vi "Simple Delay Line.vi"() -> ()   [LabVIEW 2015]
uses:
  <vilib>/DAQmx/read.llb/DAQmx Read (Analog Wfm 1Chan NSamp).vi
  <vilib>/DAQmx/write.llb/DAQmx Write (Analog Wfm 1Chan NSamp).vi
  <vilib>/DAQmx/create/channels.llb/DAQmx Create Channel (AI-Voltage-Basic).vi
  <vilib>/DAQmx/create/channels.llb/DAQmx Create Channel (AO-Voltage-Basic).vi
  <vilib>/DAQmx/configure/timing.llb/DAQmx Timing (Sample Clock).vi
  <vilib>/DAQmx/configure/trigger.llb/DAQmx Reference Trigger (Analog Window).vi
  <vilib>/DAQmx/miscellaneous.llb/DAQmx Fill In Error Info.vi
  <resource>/objmgr/daqmx.rc
panel:
  in  "Speaker IR":path
  in  "Stimuli":dbl[](array[numeric])
  in  "Stimulus File":path=path "C:/Kate/matlabstim/IRs/testIR.mat"
  out "Now Playing":dbl=3.0
  out "data 2":waveform(dbl)(graph) caption="Stim"
  out "data":waveform(dbl)(graph)={"t0"=timestamp(3665351973.137573 s since 1904-01-01), "dt"=3.999999999999989e-06, "Y"=array[1250 elements], "attributes"=variant("NI_ChannelName"=variant(string "PXI1Slot2/ai1"), "NI_UnitDescription"=variant(string "Volts"))} caption="Call"
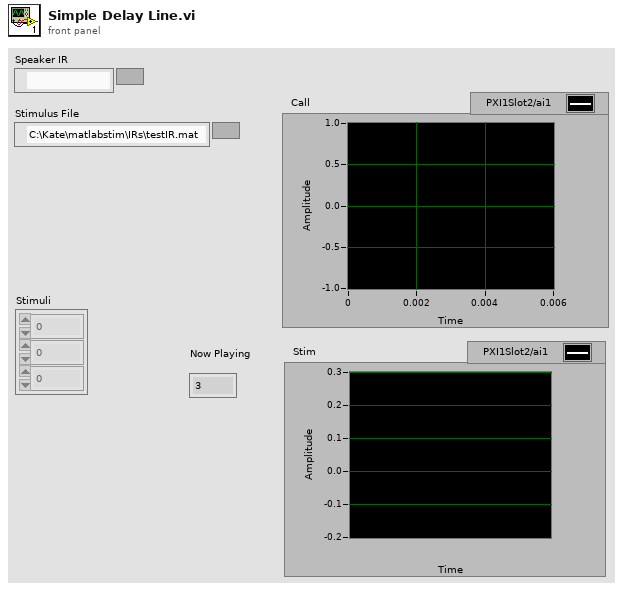
[diagram p1: front panel]
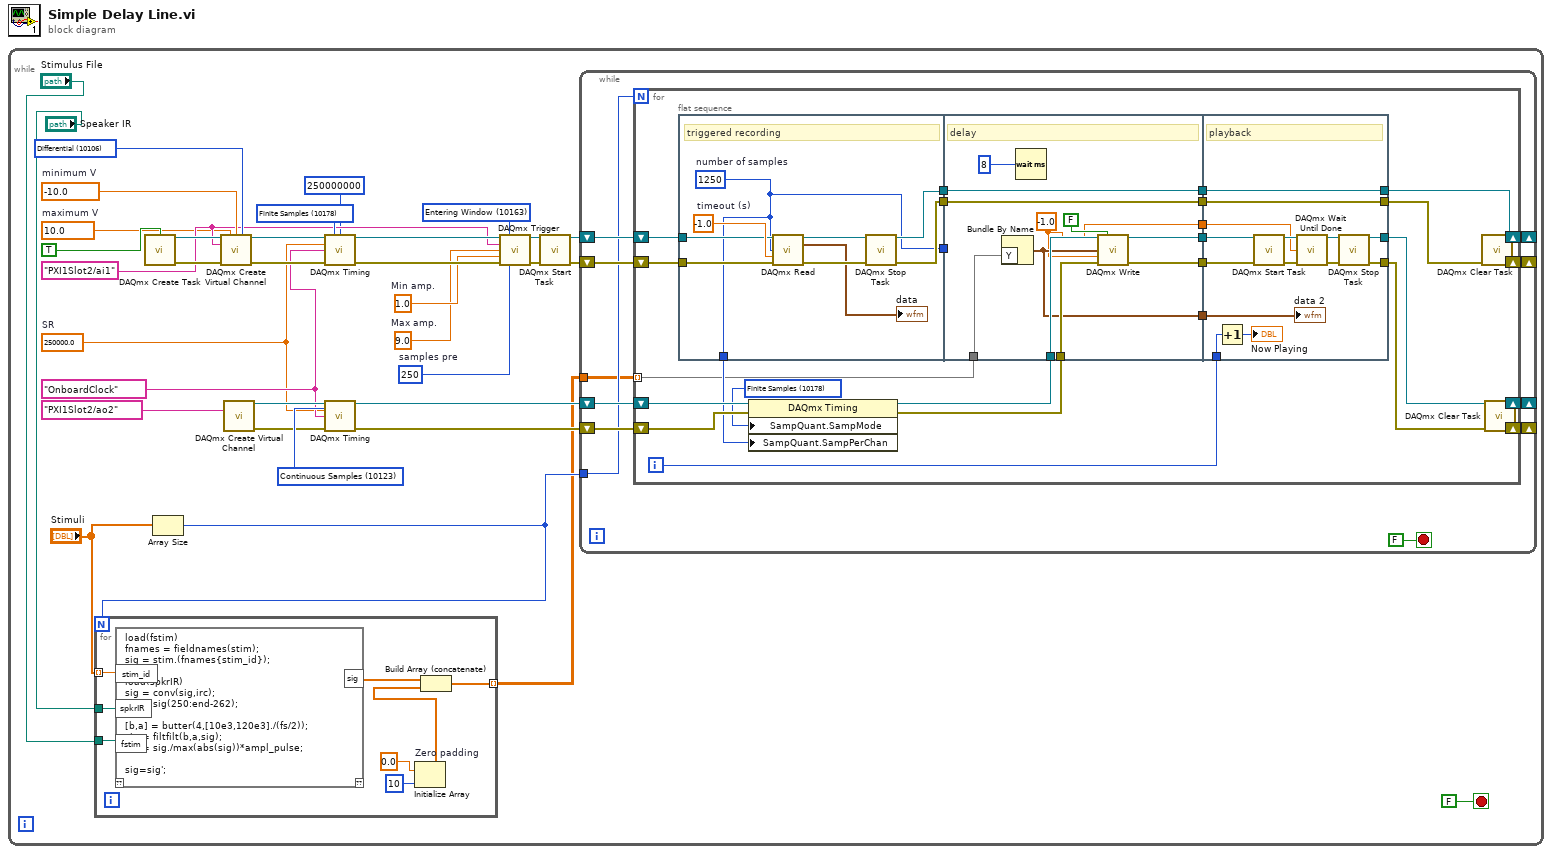
[diagram p0: block diagram]
diagram:
  n1 = while {
    stop <- FALSE stop-if-true
    w4 = tag "OnboardClock" ("source")
    w12 = 10123 items=["Finite Samples"=10178, "Continuous Samples"=10123, "Hardware Timed Single Point"=12522] ("sample mode")
    w23 = 9.0  # Max amp.
    w24 = u32 250  # samples pre
    w25 = 1.0  # Min amp.
    w26 = 10163 items=["Entering Window"=10163, "Leaving Window"=10208] ("when")
    w36 = 10106 items=["default"=-1, "RSE"=10083, "NRSE"=10078, "Differential"=10106, "Pseudodifferential"=12529] ("input terminal configuration")
    w35 = -10.0  # minimum V
    w27 = 10.0  # maximum V
    w28 = "PXI1Slot2/ai1" ("physical channel")
    w38 = 10178 items=["Finite Samples"=10178, "Continuous Samples"=10123, "Hardware Timed Single Point"=12522] ("sample mode")
    w2 = 250000.0  # SR
    n2 = call <vilib>:"DAQmx Create Task.vi"("auto cleanup"=TRUE) -> ("task out"=w32:refnum<k21>, "error out"=w31:errorcluster)  [unwired: 13 in]
    n3 = Array Size(array="Stimuli") -> (size(s)=w7:i32)
    n4 = for {
      N: w7 -> [_]
      tunnel: [w109] -> w5 mode=indexing
      tunnel: "Stimuli" -> [w115] mode=indexing
      tunnel: "Stimulus File" -> [w111]
      tunnel: "Speaker IR" -> [w108]
      n5 = script code="load(fstim)\nfnames = fieldnames(stim);\nsig = stim.(fnames{stim_id});\n\nload(spkrIR)\nsig = conv(sig,irc);\nsig = sig(250:end-262);\n\n[b,a] = butter(4,[10e3,120e3]./(fs/2));\nsig = filtfilt(b,a,sig);\nsig = sig./max(abs(sig))*ampl_pulse;\n\nsig=sig';"("stim_id"=w115, "fstim"=w111, "spkrIR"=w108) -> ("sig"=w114:dbl[])  [unwired: 1 in, 1 out]
      n6 = Initialize Array "Zero padding"(0.0, 10) -> (w113:dbl[])
      n7 = Build Array (concatenate)(w114, w113) -> (w109:dbl[])
    }
    n8 = call-poly <vilib>:"DAQmx Create Virtual Channel.vi"("task in"=w32, "maximum value"=w27, "minimum value"=w35, "input terminal configuration"=w36, "physical channels"=w28, "error in"=w31) -> ("task out"=w34:refnum<k21>, "error out"=w33:errorcluster)  [unwired: 8 in]
    n9 = call-poly <vilib>:"DAQmx Create Virtual Channel.vi"("physical channels"=tag "PXI1Slot2/ao2") -> ("task out"=w11:refnum<k21>, "error out"=w10:errorcluster)  [unwired: 13 in]
    n10 = call-poly <vilib>:"DAQmx Timing.vi"("task/channels in"=w34, "sample mode"=w38, "samples per channel"=250000000, "rate"=w2, "source"=w4, "error in"=w33) -> ("task out"=w37:refnum<k21>, "error out"=w30:errorcluster)  [unwired: 8 in]
    n11 = call-poly <vilib>:"DAQmx Timing.vi"("task/channels in"=w11, "sample mode"=w12, "rate"=w2, "source"=w4, "error in"=w10) -> ("task out"=w9:refnum<k21>, "error out"=w8:errorcluster)  [unwired: 9 in]
    n12 = call-poly <vilib>:"DAQmx Trigger.vi"("task/channels in"=w37, "when"=w26, "source"=w28, "window top"=w23, "window bottom"=w25, "error in"=w30, "pretrigger samples per channel"=w24) -> ("task out"=w20:refnum<k21>, "error out"=w19:errorcluster)  [unwired: 7 in]
    n13 = call <vilib>:"DAQmx Start Task.vi"("task/channels in"=w20, "error in"=w19) -> ("task out"=w17:refnum<k21>, "error out"=w18:errorcluster)  [unwired: 12 in]
    n14 = while {
      tunnel: w7 -> [w42]
      shift-right: [w49] -> w21
      shift-left: w18 -> [w48]
      shift-right: [w50] -> w22
      shift-left: w17 -> [w47]
      shift-right: [w46] -> w15
      shift-left: w9 -> [w44]
      shift-right: [w45] -> w14
      shift-left: w8 -> [w43]
      tunnel: w5 -> [w40]
      stop <- FALSE ("stop") stop-if-true
      n15 = for {
        N: w42 -> [_]
        shift-right: [w66] -> w49
        shift-left: w48 -> [w69]
        shift-right: [w67] -> w50
        shift-left: w47 -> [w68]
        shift-right: [w65] -> w46
        shift-left: w44 -> [w64]
        shift-right: [w63] -> w45
        shift-left: w43 -> [w62]
        tunnel: w40 -> [w51] mode=indexing
        i -> [w60]
        w61 = 10178 items=["Finite Samples"=10178, "Continuous Samples"=10123, "Hardware Timed Single Point"=12522] ("SampQuant.SampMode")
        n16 = flat-sequence {
          tunnel: [w77] -> w73
          tunnel: [w76] -> w72
          tunnel: w69 -> [w79]
          tunnel: w68 -> [w78]
          tunnel: [w74] -> w52
          tunnel: [w74] -> w54
          tunnel: w73 -> [w93]
          tunnel: [w93] -> w71
          tunnel: w72 -> [w92]
          tunnel: [w92] -> w70
          tunnel: w59 -> [w89]
          tunnel: w58 -> [w88]
          tunnel: [w87] -> w57
          tunnel: [w86] -> w56
          tunnel: [w85] -> w55
          tunnel: w54 -> [_]
          tunnel: [w84] -> w53
          tunnel: w51 -> [w83]
          tunnel: [w102] -> w65
          tunnel: w71 -> [w107]
          tunnel: w70 -> [w106]
          tunnel: [w107] -> w67
          tunnel: [w106] -> w66
          tunnel: [w103] -> w63
          tunnel: w60 -> [w98]
          tunnel: w57 -> [w97]
          tunnel: w56 -> [w96]
          tunnel: w55 -> [w95]
          tunnel: w53 -> [w94]
          frame #0 {
            w74 = 1250  # number of samples
            w81 = -1.0  # timeout (s)
            # "triggered recording"
            n17 = call-poly <vilib>:"DAQmx Read.vi"("task/channels in"=w78, "number of samples per channel"=w74, "timeout"=w81, "error in"=w79) -> ("task out"=w82:refnum<k21>, "data"=→"data":waveform(dbl), "error out"=w80:errorcluster)  [unwired: 9 in]
            n18 = call <vilib>:"DAQmx Stop Task.vi"("task/channels in"=w82, "error in"=w80) -> ("task out"=w77:refnum<k21>, "error out"=w76:errorcluster)  [unwired: 12 in]
          }
          frame #1 {
            w84 = -1.0 ("timeout")
            # "delay"
            n19 = Bundle By Name("Y"=w83) -> (w85:waveform(dbl))  [unwired: 1 in]
            n20 = Wait (ms)(milliseconds to wait=8) -> ()  [unwired: 1 out]
            n21 = call-poly <vilib>:"DAQmx Write.vi"("task/channels in"=w89, "auto start"=FALSE, "data"=w85, "timeout"=w84, "error in"=w88) -> ("task out"=w87:refnum<k21>, "error out"=w86:errorcluster)  [unwired: 8 in, 1 out]
          }
          frame #2 {
            # "playback"
            n22 = Increment(x=w98) -> (x+1=→"Now Playing":i32)
            n23 = call <vilib>:"DAQmx Start Task.vi"("task/channels in"=w97, "error in"=w96) -> ("task out"=w100:refnum<k21>, "error out"=w99:errorcluster)  [unwired: 12 in]
            n24 = call <vilib>:"DAQmx Wait Until Done.vi"("task/channels in"=w100, "timeout (sec)"=w94, "error in"=w99) -> ("task out"=w105:refnum<k21>, "error out"=w104:errorcluster)  [unwired: 11 in]
            n25 = call <vilib>:"DAQmx Stop Task.vi"("task/channels in"=w105, "error in"=w104) -> ("task out"=w102:refnum<k21>, "error out"=w103:errorcluster)  [unwired: 12 in]
            "data 2" <- w95
          }
        }
        n26 = property class="DAQmx Timing"(reference=w64, error in=w62, "SampQuant.SampMode"=w61, "SampQuant.SampPerChan"=w52) -> (reference out=w59:refnum<k21>, error out=w58:errorcluster)
      }
    }
    n27 = call <vilib>:"DAQmx Clear Task.vi"("task in"=w22, "error in"=w21) -> ()  [unwired: 13 in, 1 out]
    n28 = call <vilib>:"DAQmx Clear Task.vi"("task in"=w15, "error in"=w14) -> ()  [unwired: 13 in, 1 out]
  }
